vi "Create lvlib Folder.vi"(9 "Name":string, 10 "Project:Active Project":refnum<vi>) -> (2 "Library Folder Path":path)   [LabVIEW 2021, in "_Template.lvlib" / "Script Strategy.lvlib"]
uses:
  Script Strategy.lvlib
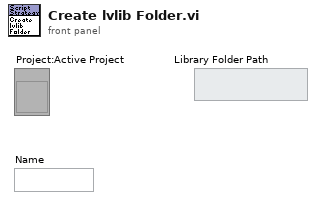
[diagram p1: front panel]
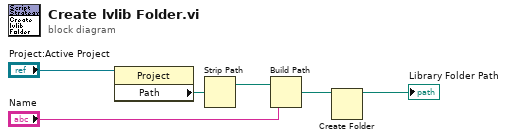
[diagram p0: block diagram]
diagram:
  n1 = property class="Project"(reference="Project:Active Project") -> ("Path"=w4:path)  [unwired: 1 in, 2 out]
  n2 = Strip Path(path=w4) -> (stripped path=w5:path)  [unwired: 1 out]
  n3 = Build Path(base path=w5, name or relative path="Name") -> (appended path=w6:path)
  n4 = Create Folder(path (use dialog)=w6) -> (created path=→"Library Folder Path":path)  [unwired: 2 in, 2 out]
